vi "Read Sweep Configuration File.vi"(8 "error in (no error)":errorcluster, 10 "Path":path, 11 "SweepControl in":refnum<class "Sweep Control.lvclass">) -> (0 "error out":errorcluster, 2 "Data":variant, 3 "SweepControl out":refnum<class "Sweep Control.lvclass">)   [LabVIEW 2019, in "Sweep Control.lvclass"]
uses:
  Sweep Control.lvclass
  Typedefs/Enum - Experiments.ctl
  Typedefs/Continuous B Sweep JSON--Cluster.ctl
  Typedefs/Enum - Priority.ctl
  Typedefs/Enum - Action.ctl
  Typedefs/Cluster - ScanControl.ctl
  Typedefs/ScanControl.ctl
  Typedefs/Cluster - ScanParamters.ctl
  Typedefs/ScanParamters.ctl
  Typedefs/Sweep Control JSON--Cluster.ctl
  <vilib>/addons/_JKI.lib/Serialization/JSON/JKI JSON Serialization.lvlib
  <userlib>/LevyLab/Krohn Hite 7008/typedefs/Input Configuration-Enum.ctl
  <userlib>/LevyLab/Krohn Hite 7008/Instrument.KH7008.lvclass
  <userlib>/LevyLab/Krohn Hite 7008/typedefs/Shunt-Enum.ctl
  <userlib>/LevyLab/Krohn Hite 7008/typedefs/Gain-Enum.ctl
  <userlib>/LevyLab/Krohn Hite 7008/typedefs/Channel-Enum.ctl
  <userlib>/LevyLab/Transport/Typedefs/Wiring Description--cluster.ctl
  <userlib>/LevyLab/Transport/Control Experiment.lvclass
  <userlib>/LevyLab/Transport/Typedefs/Instrument--enum.ctl
  <userlib>/LevyLab/Transport/Typedefs/Experiment Description--cluster.ctl
  <userlib>/LevyLab/Transport/Typedefs/Lockin_Sweep JSON--Cluster.ctl
  <userlib>/LevyLab/Transport/Transport.lvclass
  <userlib>/LevyLab/Krohn Hite 7008/typedefs/Coupling-Enum.ctl
  <userlib>/LevyLab/Krohn Hite 7008/typedefs/Filter-Enum.ctl
  <userlib>/LevyLab/Krohn Hite 7008/typedefs/SetAll-Cluster.ctl
  <userlib>/LevyLab/Krohn Hite 7008/typedefs/SetAll-Array.ctl
  <userlib>/LevyLab/Transport/Typedefs/Instrument Types--combo.ctl
  <userlib>/LevyLab/Lockin-Multichannel/Instrument.DAQ/Typedefs/REF.Channel--Cluster.ctl
  <userlib>/LevyLab/Lockin-Multichannel/Instrument.DAQ/Instrument.DAQ.lvclass
  <userlib>/LevyLab/Lockin-Multichannel/Instrument.DAQ/Typedefs/REF.Channel--Cluster--Array.ctl
  <userlib>/LevyLab/Lockin-Multichannel/Instrument.DAQ/Typedefs/AO.Channel.Function--Enum.ctl
  <userlib>/LevyLab/Lockin-Multichannel/Instrument.DAQ/Typedefs/AO.Channel--Cluster.ctl
  <userlib>/LevyLab/Lockin-Multichannel/Instrument.DAQ/Typedefs/AO.Channel--Cluster--Array.ctl
  <userlib>/LevyLab/Lockin-Multichannel/Instrument.DAQ/Typedefs/Sweep.Pattern--Enum.ctl
  <userlib>/LevyLab/Lockin-Multichannel/Instrument.DAQ/Typedefs/Sweep.Channel--Cluster.ctl
  <userlib>/LevyLab/Lockin-Multichannel/Instrument.DAQ/Typedefs/Sweep.Channel--Cluster--Array.ctl
  <userlib>/LevyLab/Transport/Typedefs/Instruments--cluster.ctl
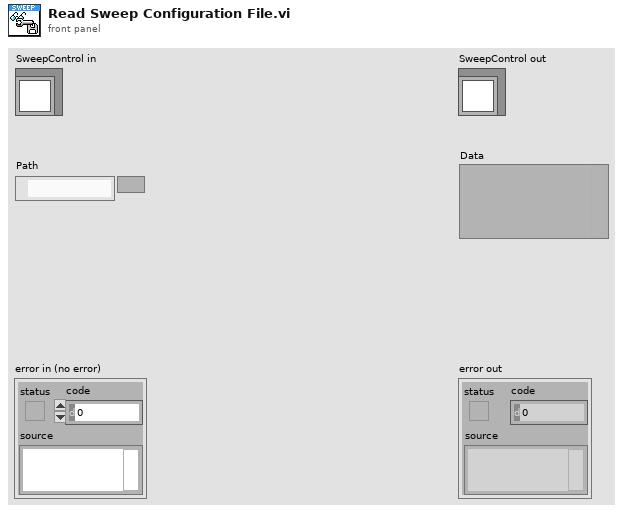
[diagram p1: front panel]
types:
  T1 = typedef "Transport.lvclass/Lockin_Sweep JSON--Cluster.ctl" = cluster{"Sweep Time (s)":dbl, "Initial Wait (s)":dbl, "Return to Start":bool, "Sweep Channels":T2, "Sweep Tables":cluster{"Ch":i32, "Table":dbl[]}[]}
  T2 = typedef "Instrument.DAQ.lvclass/Sweep.Channel--Cluster--Array.ctl" = T3[]
  T3 = typedef "Instrument.DAQ.lvclass/Sweep.Channel--Cluster.ctl" = cluster{"Enable?":bool, "Channel":u16, "Start":dbl, "End":dbl, "Pattern":T4, "Table":dbl[]}
  T4 = typedef "Instrument.DAQ.lvclass/Sweep.Pattern--Enum.ctl" = enum16{"Ramp /", "Ramp /\\", "Smooth Ramp _/", "Smooth Ramp _/\\_", "Table"}
  T5 = typedef "Sweep Control.lvclass/Continuous B Sweep JSON--Cluster.ctl" = cluster{"Continuous B Sweep":cluster{"Experiment":T6, "B field values":dbl[]}, "Experiment Description":T7, "Wiring Configuration":T11, "Lockin":cluster{"AOconfig":T12, "REFconfig":T15}, "Krohn Hite":cluster{"Channel Setting":T17}}
  T6 = typedef "Sweep Control.lvclass/Enum - Experiments.ctl" = enum16{"Lockin_time", "Lockin_sweep", "Lockin_DelayLine"}
  T7 = typedef "Control Experiment.lvclass/Experiment Description--cluster.ctl" = cluster{"User":string, "Device":string, "Device Path":path, "Device Description":string, "Experiment Path":path, "Experiment Description":string, "Instrument":T8, "Instruments":T9[], "Sweep":cluster{"key":string, "value":variant}[]}
  T8 = typedef "Control Experiment.lvclass/Instrument--enum.ctl" = enum16{"----- AFM/EBL -----", "AGILENT", "CYPHER", "Gemini2", "JEOL", "MFP3D", "----- Cryostat -----", "CF900", "DR200", "MNK", "PPMS (simulated)", "PPMS 1", "PPMS 2", "PPMS 3", "----- Optics -----", "THz 1 (Element 2/Montana)", "THz 2 (Tsunami/Janis)"}
  T9 = typedef "Control Experiment.lvclass/Instruments--cluster.ctl" = cluster{"class path":path, "Address":string, "Type":T10}
  T10 = typedef "Control Experiment.lvclass/Instrument Types--combo.ctl" = string
  T11 = typedef "Control Experiment.lvclass/Wiring Description--cluster.ctl" = cluster{"Lockin Ch":i32[], "KH":cluster{"Electrodes":string[], "Labels":string[]}, "not KH":cluster{"Electrodes":string[], "Labels":string[]}}
  T12 = typedef "Instrument.DAQ.lvclass/AO.Channel--Cluster--Array.ctl" = T13[]
  T13 = typedef "Instrument.DAQ.lvclass/AO.Channel--Cluster.ctl" = cluster{"Enable?":bool, "Channel":i32, "Amplitude":dbl, "Offset":dbl, "Frequency":dbl, "Phase":dbl, "Function":T14, "Sweeping?":bool}
  T14 = typedef "Instrument.DAQ.lvclass/AO.Channel.Function--Enum.ctl" = enum16{"Sine", "Triangle", "Square"}
  T15 = typedef "Instrument.DAQ.lvclass/REF.Channel--Cluster--Array.ctl" = T16[]
  T16 = typedef "Instrument.DAQ.lvclass/REF.Channel--Cluster.ctl" = cluster{"Enable?":bool, "Channel":i32, "Frequency":dbl, "Phase":dbl, "TC":dbl, "Roll-Off":i32}
  T17 = typedef "Instrument.KH7008.lvclass/SetAll-Array.ctl" = T18[]
  T18 = typedef "Instrument.KH7008.lvclass/SetAll-Cluster.ctl" = cluster{"Channel":T19, "Gain":T20, "Bandwidth Filter":T21, "Shunt Resistor":T22, "Coupling":T23, "Input Config":T24}
  T19 = typedef "Instrument.KH7008.lvclass/Channel-Enum.ctl" = enum16{"Channel 1", "Channel 2", "Channel 3", "Channel 4", "Channel 5", "Channel 6", "Channel 7", "Channel 8"}
  T20 = typedef "Instrument.KH7008.lvclass/Gain-Enum.ctl" = enum16{"1x", "10x", "100x", "1000x"}
  T21 = typedef "Instrument.KH7008.lvclass/Filter-Enum.ctl" = enum16{"OFF", "ON"}
  T22 = typedef "Instrument.KH7008.lvclass/Shunt-Enum.ctl" = enum16{"Open", "50 Ohms", "500 Ohms", "5k Ohms", "50k Ohms", "10M Ohm"}
  T23 = typedef "Instrument.KH7008.lvclass/Coupling-Enum.ctl" = enum16{"AC", "DC"}
  T24 = typedef "Instrument.KH7008.lvclass/Input Configuration-Enum.ctl" = enum16{"Ground", "SE+ (-gnd)", "SE- (+gnd)", "Differential"}
  T25 = typedef "Sweep Control.lvclass/Sweep Control JSON--Cluster.ctl" = cluster{"Experiment":T6, "Repeat Experiment":i32, "Scan control":T26, "Scan parameters":T30}
  T26 = typedef "Sweep Control.lvclass/ScanControl.ctl" = T27[]
  T27 = typedef "Sweep Control.lvclass/Cluster - ScanControl.ctl" = cluster{"Priority":T28, "Scan name":T29}
  T28 = typedef "Sweep Control.lvclass/Enum - Priority.ctl" = enum16{"Priority 0", "Priority 1", "Priority 2", "Priority 3", "Priority 4", "Priority 5"}
  T29 = typedef "Sweep Control.lvclass/Enum - Action.ctl" = enum16{"OFF", "time", "Lockin Amplitude", "Lockin Frequency", "Lockin Bias", "Delay", "Strain", "DAQ Bias", "Magnet Field", "Temperature", "MW f1", "MW f2", "MW Amplitude1", "MW Amplitude2"}
  T30 = typedef "Sweep Control.lvclass/ScanParamters.ctl" = T31[]
  T31 = typedef "Sweep Control.lvclass/Cluster - ScanParamters.ctl" = cluster{"Start":dbl, "End":dbl, "Step":dbl, "Rate":dbl, "Waveform type":enum16{"linear", "triangle", "power"}, "wait (ms or K)":dbl, "Address":string, "channel":i32}
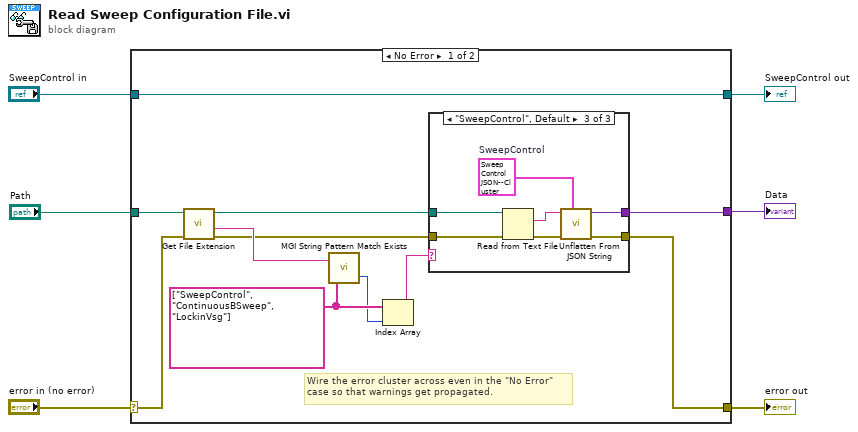
[diagram p0: block diagram]
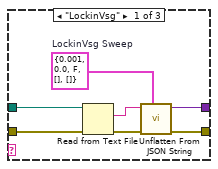
[diagram p2: hidden frame]
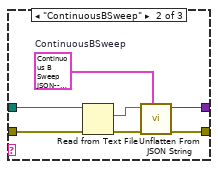
[diagram p3: hidden frame]
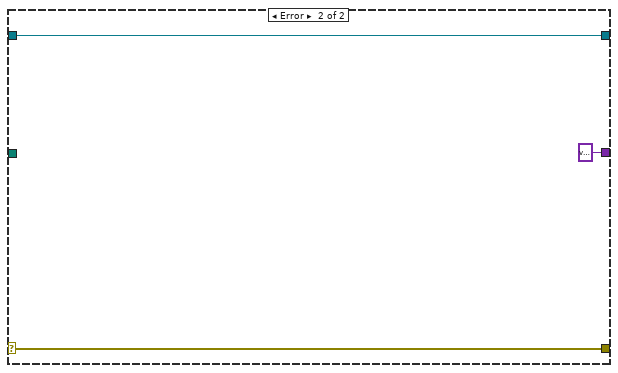
[diagram p4: hidden frame]
diagram:
  n1 = case shown="No Error" "error in (no error)" {
    selector: "error in (no error)" -> [w8 w41]
    tunnel: [w7 w41] -> w5
    tunnel: [w17 w40] -> w3
    tunnel: "SweepControl in" -> [w17 w40]
    tunnel: "Path" -> [w16 _]
    tunnel: [w9 variant ("Variant")] -> w1
    frame No Error {
      w14 = string[] ["SweepControl", "ContinuousBSweep", "LockinVsg"] ("Patterns to Try")
      # "Wire the error cluster across even in the \"No Error\"\ncase so that warnings get propagated."
      n2 = call <vilib>:"Get File Extension.vi"("error in (no error)"=w8, "file"=w16) -> ("error out"=w11:errorcluster, "filename without extension"=w13:string, "dup file"=w10:path)  [unwired: 5 in, 2 out]
      n3 = call <userlib>:"MGI String Pattern Match Exists.vi"("Patterns to Try"=w14, "String"=w13) -> ("Index of First Pattern Matched"=w12:i32)  [unwired: 1 out]
      n4 = Index Array(array=w14, index=w12) -> (element=w15:string)
      n5 = case shown="\"SweepControl\", Default" w15 {
        tunnel: w11 -> [w22 w29 w36]
        tunnel: w10 -> [w21 w28 w35]
        tunnel: [w19 w27 w34] -> w9
        tunnel: [w18 w26 w33] -> w7
        frame "LockinVsg" {
          w20 = T1 {"Sweep Time (s)"=0.001, "Initial Wait (s)"=0.0, "Return to Start"=FALSE, "Sweep Channels"=[], "Sweep Tables"=[]}  # LockinVsg Sweep
          n6 = Read from Text File(file (use dialog)=w21, error in=w22) -> (text=w23:string, error out=w24:errorcluster)  [unwired: 2 in, 2 out]
          n7 = call <vilib>:"Unflatten From JSON String.vi"("Type and Defaults"=w20, "error in (no error)"=w24, "JSON String"=w23) -> ("error out"=w18:errorcluster, "Variant"=w19:variant)  [unwired: 7 in]
        }
        frame "ContinuousBSweep" {
          w25 = T5 {"Continuous B Sweep"={"Experiment"=enum."Lockin_DelayLine", "B field values"=[]}, "Experiment Description"={"User"="", "Device"="", "Device Path"=path "", "Device Description"="", "Experiment Path"=path "", "Experiment Description"="", "Instrument"=enum."PPMS 1", "Instruments"=[], "Sweep"=[]}, "Wiring Configuration"={"Lockin Ch"=[], "KH"={"Electrodes"=[], "Labels"=[]}, "not KH"={"Electrodes"=[], "Labels"=[]}}, "Lockin"={"AOconfig"=[], "REFconfig"=[]}, "Krohn Hite"={"Channel Setting"=[]}}  # ContinuousBSweep
          n8 = Read from Text File(file (use dialog)=w28, error in=w29) -> (text=w30:string, error out=w31:errorcluster)  [unwired: 2 in, 2 out]
          n9 = call <vilib>:"Unflatten From JSON String.vi"("Type and Defaults"=w25, "error in (no error)"=w31, "JSON String"=w30) -> ("error out"=w26:errorcluster, "Variant"=w27:variant)  [unwired: 7 in]
        }
        frame "SweepControl", Default {
          w32 = T25 {"Experiment"=enum."Lockin_DelayLine", "Repeat Experiment"=0, "Scan control"=[], "Scan parameters"=[]}  # SweepControl
          n10 = Read from Text File(file (use dialog)=w35, error in=w36) -> (text=w37:string, error out=w38:errorcluster)  [unwired: 2 in, 2 out]
          n11 = call <vilib>:"Unflatten From JSON String.vi"("Type and Defaults"=w32, "error in (no error)"=w38, "JSON String"=w37) -> ("error out"=w33:errorcluster, "Variant"=w34:variant)  [unwired: 7 in]
        }
      }
    }
    frame Error {
    }
  }
  "error out" <- w5
  "SweepControl out" <- w3
  "Data" <- w1
